vi "Record Analog Info.vi"(1 "input limits (no change)":T1(array[cluster]) {"low limit (-10V)" format="%.2f"; "high limit (10V)" format="%.2f"}, 2 "channels (0)":i32[](array[numeric]), 3 "Boolean":bool, 4 "File Ref Num 2":refnum<file>) -> (0 "File Ref Num":refnum<file>)   [LabVIEW 2021]
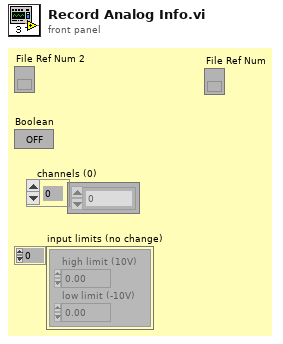
[diagram p1: front panel]
types:
  T1 = cluster{"high limit (10V)":sgl, "low limit (-10V)":sgl}[]
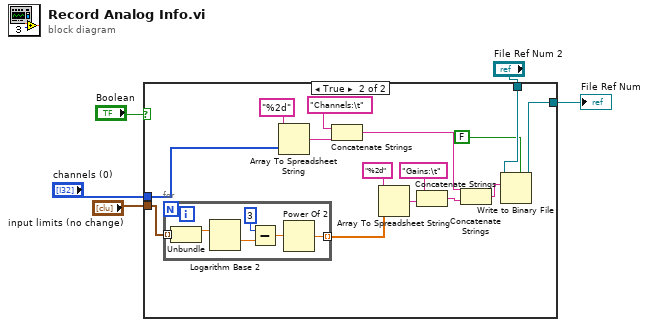
[diagram p0: block diagram]
diagram:
  n1 = case shown="True" "Boolean" {
    tunnel: "channels (0)" -> [_ w12]
    tunnel: "input limits (no change)" -> [_ w10]
    tunnel: "File Ref Num 2" -> [w6 w11]
    tunnel: [w6 w8] -> w5
    frame False {
    }
    frame True {
      n2 = for {
        tunnel: w10 -> [w27] mode=indexing
        tunnel: [w22] -> w9 mode=indexing
        n3 = Unbundle(w27) -> ("high limit (10V)"=w26:sgl)  [unwired: 1 out]
        n4 = Logarithm Base 2(1:w26) -> (0:w25:sgl)
        n5 = Subtract(x=3, y=w25) -> (x-y=w23:sgl)
        n6 = Power Of 2(x=w23) -> (2^x=w22:sgl)
      }
      n7 = Array To Spreadsheet String(array=w12, 3:"%2d") -> (spreadsheet string=w13:string)  [unwired: 1 in]
      n8 = Concatenate Strings("Channels:\t", w13) -> (w20:string)
      n9 = Array To Spreadsheet String(array=w9, 3:"%2d") -> (spreadsheet string=w18:string)  [unwired: 1 in]
      n10 = Concatenate Strings("Gains:\t", w18) -> (w21:string)
      n11 = Concatenate Strings(w20, w21) -> (w16:string)
      n12 = Write to Binary File(file (use dialog)=w11, data=w16, 5:FALSE ("prepend array or string size? (T)")) -> (refnum out=w8:refnum<file>)  [unwired: 3 in, 2 out]
    }
  }
  "File Ref Num" <- w5
